vi "Z Aux Flash Readf.vi"(0 "handle":u32, 1 "puinumesread":u32, 5 "uiflashid":u16, 7 "uibuffnum":u32, 9 "pfvlue":sgl[](array[numeric])=array[4097 elements], 11 "error in (no error)":errorcluster caption="错误输入（无错误）") -> (3 "puinumesread out":u32, 4 "handle out":u32, 6 "function return":i32, 10 "pfvlue out":sgl[](array[numeric]), 15 "error out":errorcluster caption="错误输出")   [LabVIEW 2015, in "zauxdll.lvlib"]
doc: "int32 __stdcall ZAux_FlashReadf(ZMC_HANDLE handle, uint16 uiflashid, uint32 uibuffnum, float pfvlue[], uint32* puinumesread);"
uses:
  zauxdll.lvlib
  Radar - 2015 32bit_autoqueue_angle_0319/zauxdll-2014/zauxdll.dll
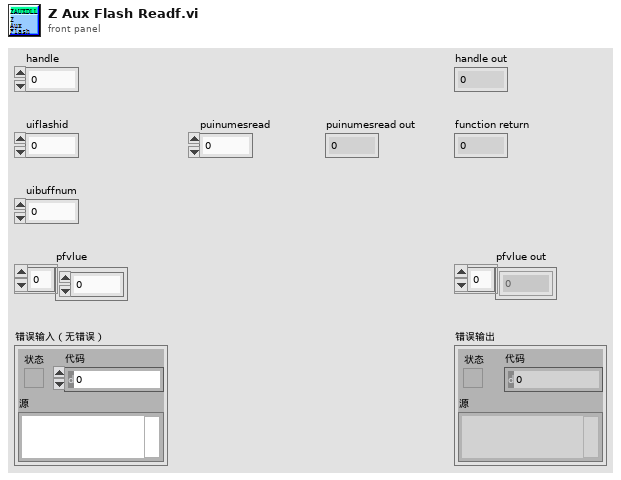
[diagram p1: front panel]
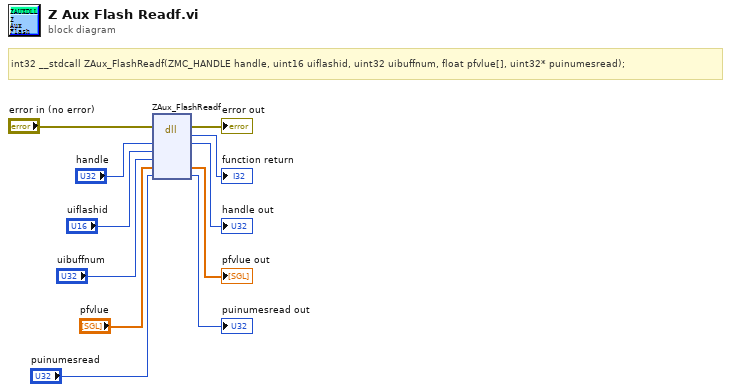
[diagram p0: block diagram]
diagram:
  # "int32 __stdcall ZAux_FlashReadf(ZMC_HANDLE handle, uint16 uiflashid, uint32 uibuffnum, float pfvlue[], uint32* puinumesread);"
  n1 = dll-call lib="D:/vicomm case/cub/0717/Radar - 2015 32bit_autoqueue_angle_0319/zauxdll-2014/zauxdll.*" fn="ZAux_FlashReadf"(error in="error in (no error)", "handle"="handle", "uiflashid"="uiflashid", "uibuffnum"="uibuffnum", "pfvlue"="pfvlue", "puinumesread"="puinumesread") -> (error out=→"error out":errorcluster, →"function return":i32, "handle"=→"handle out":u32, "pfvlue"=→"pfvlue out":sgl[], "puinumesread"=→"puinumesread out":u32)  [unwired: 4 in, 1 out]
